vi "Read String Array (1D).vi"(8 "error in":errorcluster, 11 "String Array (1D) Ref in":refnum<vi>) -> (0 "error out":errorcluster, 1 "Value":string[](array[string]), 2 "Interpret As Unicode":bool, 3 "String Array (1D) Ref out":refnum<vi>)   [LabVIEW 2020, in "G-Unicode.lvlib"]
uses:
  G-Unicode.lvlib
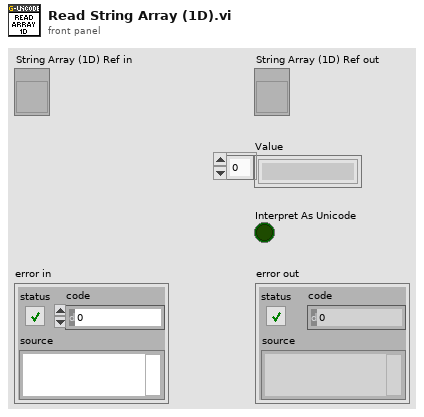
[diagram p1: front panel]
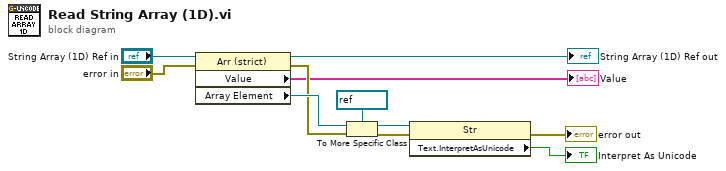
[diagram p0: block diagram]
diagram:
  n1 = property class="Arr (strict)"(reference="String Array (1D) Ref in", error in="error in") -> (reference out=→"String Array (1D) Ref out":refnum<vi>, error out=w9:errorcluster, "Value"=→"Value":string[], "Array Element"=w10:refnum<vi>)
  n2 = To More Specific Class(target class=refnum<vi> refnum ("String"), reference=w10, error in=w9) -> (specific class reference=w8:refnum<vi>, error out=w2:errorcluster)
  n3 = property class="Str"(reference=w8, error in=w2) -> (error out=→"error out":errorcluster, "Text.InterpretAsUnicode"=→"Interpret As Unicode":bool)  [unwired: 1 out]
